vi "Result_Test.vi"(8 "error in (no error)":errorcluster caption="entrée d'erreur (pas d'erreur)", 11 "Flash_Jlink en entrée":refnum<class "P2265_Boot_FW.lvclass">) -> (0 "error out":errorcluster caption="sortie d'erreur", 3 "Flash_Jlink en sortie":refnum<class "P2265_Boot_FW.lvclass">)   [LabVIEW 2020, in "Library Test.lvlib" / "P2265_Boot_FW.lvclass"]
uses:
  P2265_Boot_FW.lvclass
  C:/Users/ngarcin/OneDrive - Altyor/Standard TB/Class/Test/Test (Default)/Test (Default).lvclass
  JSON API/JSON Value/Set from JSON string.vi
  JSON API/JSON Value/JSON Value.lvclass
  Test_Without_Instr/Test_Without_Inst.lvclass
  P2265_Boot_FW.lvclass/P2265_Boot_FW.ctl
  JSON API/Variant JSON/Variant JSON.lvlib
  JSON API/Get Polymorphic/JSON GetSet.lvlib
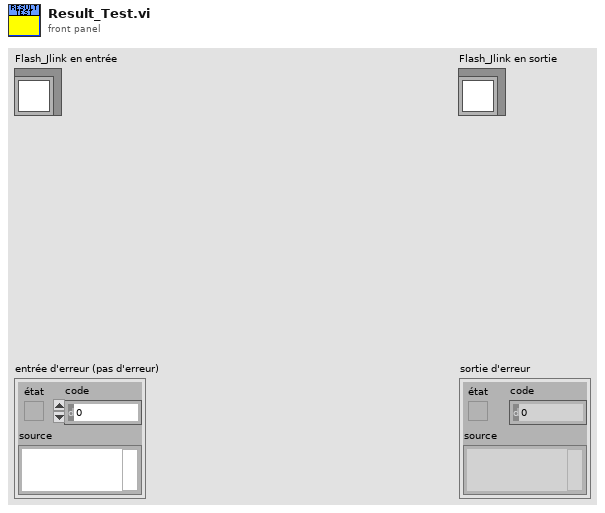
[diagram p1: front panel]
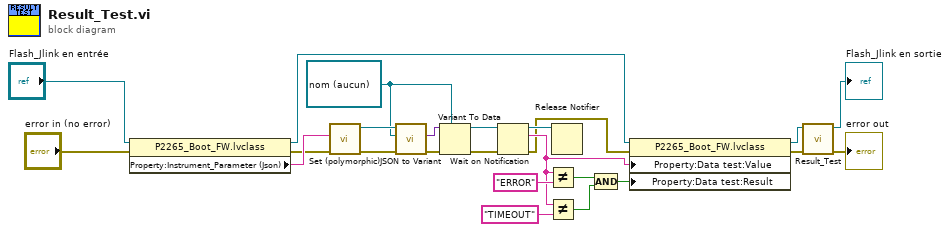
[diagram p0: block diagram]
diagram:
  w14 = refnum<notifier> refnum ("notificateur en sortie")
  n1 = property class="P2265_Boot_FW.lvclass"(reference="Flash_Jlink en entrée", error in="error in (no error)") -> (reference out=w7:refnum<class "P2265_Boot_FW.lvclass">, error out=w10:errorcluster, "Property:Instrument_Parameter (Json)"=w11:string)
  n2 = call-poly "Set (polymorphic).vi"("error in (no error)"=w10, "JSON stream"=w11) -> ("error out"=w16:errorcluster, "JSON Value out"=w18:refnum<class "JSON Value.lvclass">)  [unwired: 7 in, 1 out]
  n3 = call "JSON to Variant.vi"("error in (no error)"=w16, "Variant (Data Type)"=w14, "JSON Value"=w18) -> ("error out"=w17:errorcluster, "Variant out"=w15:variant)  [unwired: 7 in]
  n4 = Variant To Data(error in=w17, type=w14, Variant=w15) -> (data=w4:refnum<notifier>, error out=w5:errorcluster)
  n5 = Wait on Notification(notifier=w4, error in (no error)=w5) -> (notifier out=w2:refnum<notifier>, notification=w3:string, error out=w1:errorcluster)  [unwired: 2 in, 1 out]
  n6 = Not Equal?(x=w3, y="ERROR" ("expression régulière")) -> (x != y?=w21:bool)
  n7 = Not Equal?(x=w3, y="TIMEOUT" ("expression régulière")) -> (x != y?=w20:bool)
  n8 = Release Notifier(notifier=w2) -> ()  [unwired: 2 in, 3 out]
  n9 = Compound Arithmetic op=AND ("Opérateur arithmétique")(w21, w20) -> (w19:bool)
  n10 = property class="P2265_Boot_FW.lvclass"(reference=w7, error in=w1, "Property:Data test:Value"=w3, "Property:Data test:Result"=w19) -> (reference out=w6:refnum<class "P2265_Boot_FW.lvclass">, error out=w12:errorcluster)
  n11 = call-parent "Result_Test.vi"("error in (no error)"=w12, "Test_Without_Inst en entrée"=w6) -> ("error out"=→"error out":errorcluster, "Test_Without_Inst en sortie"=→"Flash_Jlink en sortie":refnum<class "P2265_Boot_FW.lvclass">)  [unwired: 8 in]
